vi "Test SaveToDisk.vi"(8 "error in (no error)":errorcluster, 11 "TestCase in":refnum<class "Verify IMemento.lvclass">) -> (0 "error out":errorcluster, 3 "TestCase out":refnum<class "Verify IMemento.lvclass">)   [LabVIEW 2009, in "Verify IMemento.lvclass"]
uses:
  Verify IMemento.lvclass
  Numeric Test Object/Interface Implementations/IMementoNumeric/MementoNumeric/MementoNumeric.lvclass
  Numeric Test Object/Numeric Test Object.lvclass
  Numeric Test Object/Interface Implementations/IMementoNumeric/IMementoNumeric.lvclass
  Framework Core/Interface Definitions/IMemento/IMemento.lvclass
  Verify IMemento.lvclass/Verify IMemento.ctl
  <vilib>/addons/_JKI Toolkits/VI Tester/TestCase.llb/TestCase.lvclass
  Source/Interfaceable Class/Interfaceable.lvclass
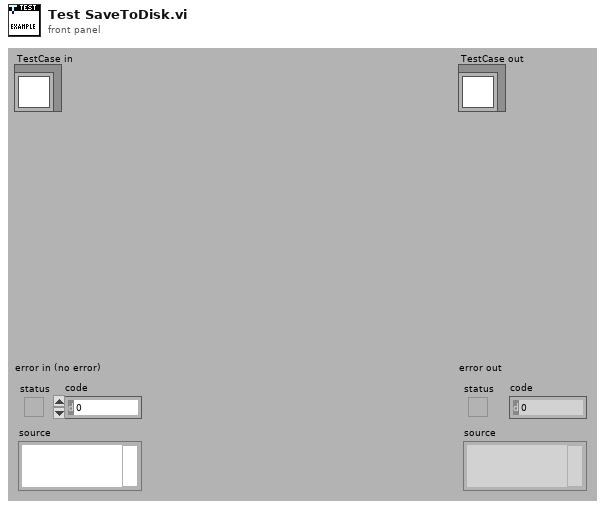
[diagram p1: front panel]
types:
  T1 = enum16{"open", "replace", "create", "open or create", "replace or create", "replace or create with confirmation"}
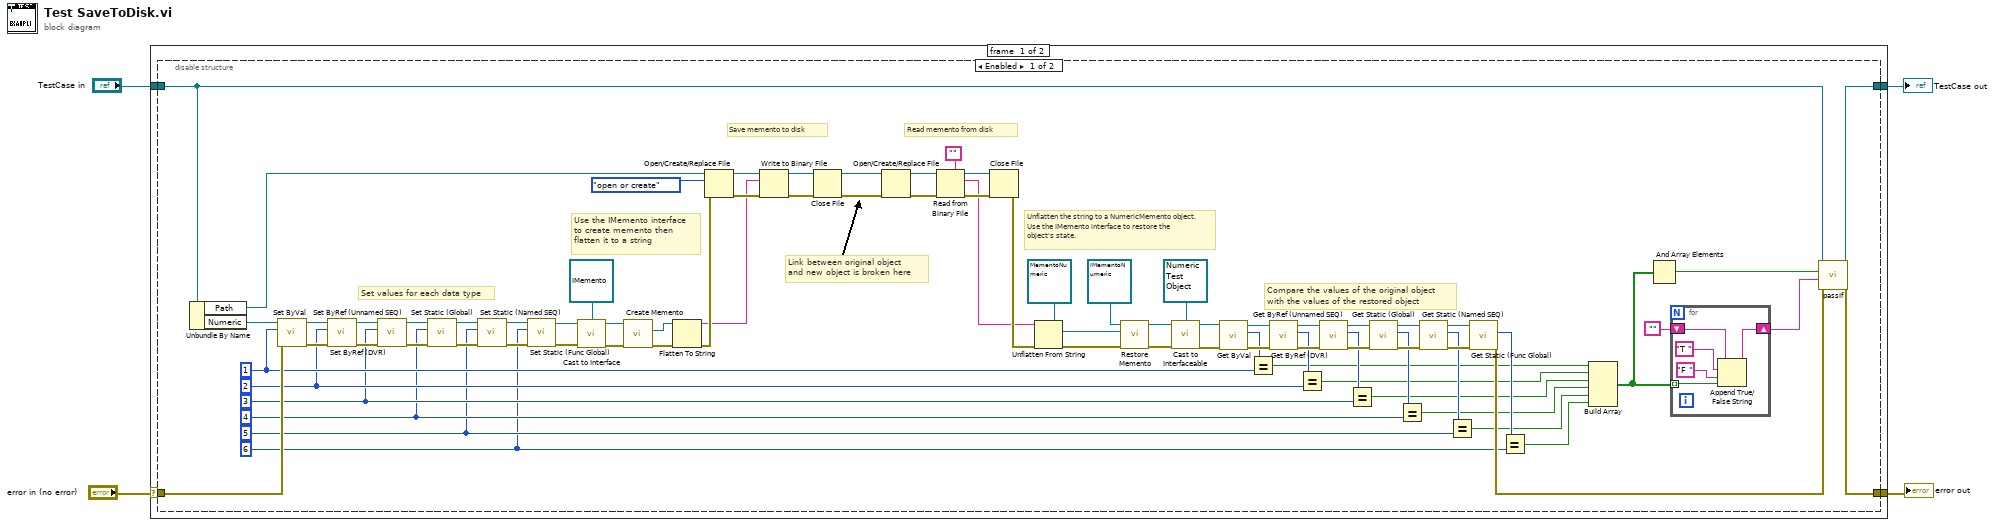
[diagram p0: block diagram]
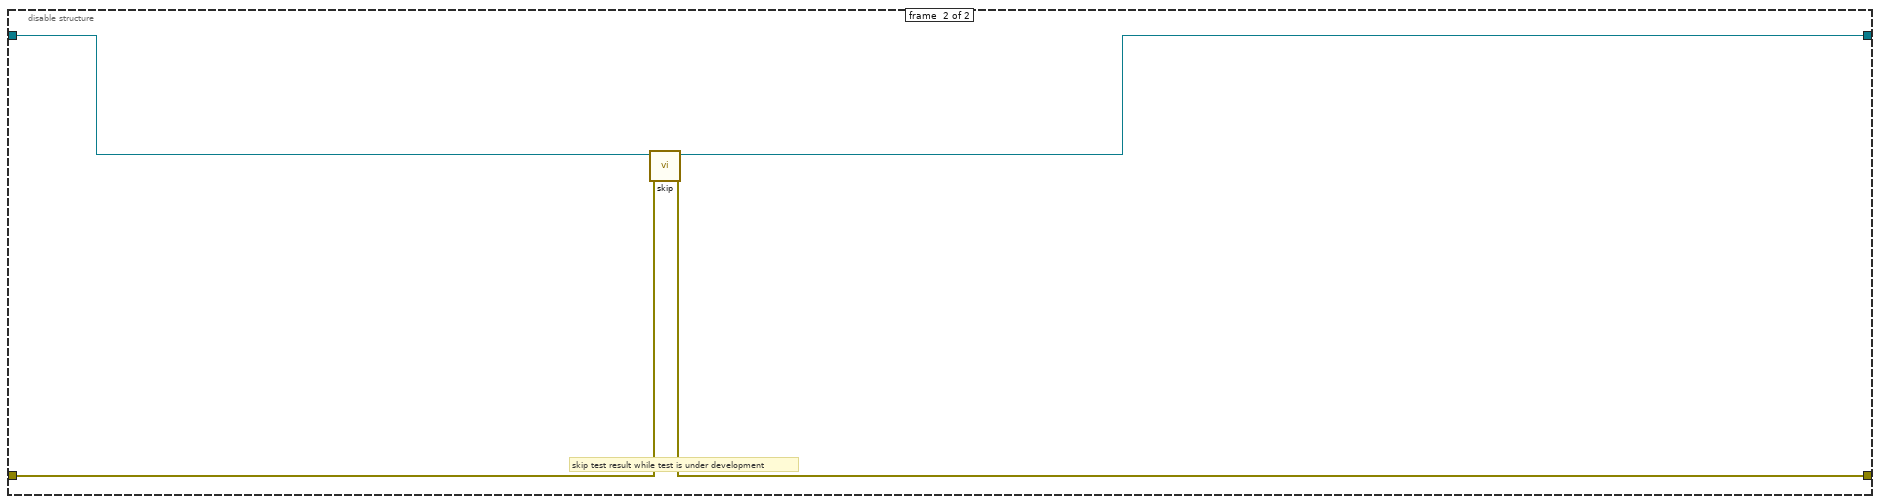
[diagram p2: hidden frame]
diagram:
  n1 = case shown="No Error" "error in (no error)" {
    selector: "error in (no error)" -> [w6 w100]
    tunnel: [w5 w100] -> w3
    tunnel: [w7 w99] -> w1
    tunnel: "TestCase in" -> [w8 w99]
    frame #0 {
      n2 = disable-structure shown="Enabled" {
        disable-tunnel: w8 -> [w66 w98]
        disable-tunnel: [w89 w95] -> w7
        disable-tunnel: w6 -> [w78 w97]
        disable-tunnel: [w88 w96] -> w5
        frame #0 {
          w29 = 1 ("Int")
          w27 = 2 ("Int")
          w25 = 3 ("Int")
          w23 = 4 ("Int")
          w21 = 5 ("Int")
          w19 = 6 ("Int")
          # "Link between original object and new object is broken here"
          # "Compare the values of the original object with the values of the restored object"
          # "Unflatten the string to a NumericMemento object. Use the IMemento interface to restore the object's state."
          # "Use the IMemento interface to create memento then flatten it to a string"
          # "Read memento from disk"
          # "Save memento to disk"
          # "Set values for each data type"
          n3 = Unbundle By Name(w66) -> ("Path"=w65:path, "Numeric"=w77:refnum<class "Numeric Test Object.lvclass">)
          n4 = call-dynamic "Set ByVal.vi"("error in (no error)"=w78, "Int"=w29, "Numeric in"=w77) -> ("error out"=w71:errorcluster, "Numeric out"=w76:refnum<class "Numeric Test Object.lvclass">)  [unwired: 7 in]
          n5 = call-dynamic "Set ByRef (DVR).vi"("error in (no error)"=w71, "Int"=w27, "Numeric in"=w76) -> ("error out"=w70:errorcluster, "Numeric out"=w75:refnum<class "Numeric Test Object.lvclass">)  [unwired: 7 in]
          n6 = call-dynamic "Set ByRef (Unnamed SEQ).vi"("error in (no error)"=w70, "Int"=w25, "Numeric in"=w75) -> ("error out"=w69:errorcluster, "Numeric out"=w74:refnum<class "Numeric Test Object.lvclass">)  [unwired: 7 in]
          n7 = call-dynamic "Set Static (Global).vi"("error in (no error)"=w69, "Int"=w23, "Numeric in"=w74) -> ("error out"=w68:errorcluster, "Numeric out"=w73:refnum<class "Numeric Test Object.lvclass">)  [unwired: 7 in]
          n8 = call-dynamic "Set Static (Named SEQ).vi"("error in (no error)"=w68, "Int"=w21, "Numeric in"=w73) -> ("error out"=w67:errorcluster, "Numeric out"=w72:refnum<class "Numeric Test Object.lvclass">)  [unwired: 7 in]
          n9 = call-dynamic "Set Static (Func Global).vi"("error in (no error)"=w67, "Int"=w19, "Numeric in"=w72) -> ("error out"=w86:errorcluster, "Numeric out"=w87:refnum<class "Numeric Test Object.lvclass">)  [unwired: 7 in]
          n10 = call "Cast to Interface.vi"("Target Interface"=refnum<class "IMemento.lvclass"> refnum ("IMemento"), "Interfaceable Object"=w87, "error in (no error)"=w86) -> ("Concrete Interface"=w84:refnum<class "IMemento.lvclass">, "error out"=w83:errorcluster)  [unwired: 5 in]
          n11 = call-dynamic "Create Memento.vi"("error in (no error)"=w83, "IMemento in"=w84) -> ("error out"=w53:errorcluster, "LabVIEW Object"=w51:refnum<class>)  [unwired: 7 in, 1 out]
          n12 = Flatten To String(anything=w51, error in (no error)=w53) -> (data string=w50:string, error out=w52:errorcluster)  [unwired: 2 in, 1 out]
          n13 = Open/Create/Replace File(file path (use dialog)=w65, error in=w52, operation (0:open)=T1."open or create") -> (refnum out=w63:refnum<file>, error out=w62:errorcluster)  [unwired: 3 in, 1 out]
          n14 = Write to Binary File(file (use dialog)=w63, data=w50, error in=w62) -> (refnum out=w61:refnum<file>, error out=w60:errorcluster)  [unwired: 3 in, 1 out]
          n15 = Close File(refnum=w61, error in=w60) -> (path=w59:path, error out=w58:errorcluster)
          n16 = Open/Create/Replace File(file path (use dialog)=w59, error in=w58) -> (refnum out=w57:refnum<file>, error out=w56:errorcluster)  [unwired: 4 in, 1 out]
          n17 = Read from Binary File(5:"" ("data type"), 8:w56, 11:w57) -> (0:w54:errorcluster, 2:w46:string, 3:w55:refnum<file>)  [unwired: 3 in, 1 out]
          n18 = Close File(refnum=w55, error in=w54) -> (error out=w48:errorcluster)  [unwired: 1 out]
          n19 = Unflatten From String(type=refnum<class "MementoNumeric.lvclass"> refnum ("MementoNumeric"), binary string=w46, error in (no error)=w48) -> (value=w43:refnum<class "MementoNumeric.lvclass">, error out=w47:errorcluster)  [unwired: 2 in, 1 out]
          n20 = call-dynamic "Restore Memento.vi"("error in (no error)"=w47, "Numeric Memento"=w43, "IMementoNumeric in"=refnum<class "IMementoNumeric.lvclass"> refnum ("IMementoNumeric")) -> ("error out"=w81:errorcluster, "IMementoNumeric out"=w82:refnum<class "IMementoNumeric.lvclass">)  [unwired: 7 in]
          n21 = call "Cast to Interfaceable.vi"("Target Object"=refnum<class "Numeric Test Object.lvclass"> refnum ("Numeric"), "Interface"=w82, "error in (no error)"=w81) -> ("Interfaceable Object"=w42:refnum<class "Numeric Test Object.lvclass">, "error out"=w41:errorcluster)  [unwired: 5 in]
          n22 = call-dynamic "Get ByVal.vi"("error in (no error)"=w41, "Numeric in"=w42) -> ("error out"=w35:errorcluster, "Int"=w30:i32, "Numeric out"=w40:refnum<class "Numeric Test Object.lvclass">)  [unwired: 7 in]
          n23 = Equal?(x=w30, y=w29) -> (x = y?=w18:bool)
          n24 = call-dynamic "Get ByRef (DVR).vi"("error in (no error)"=w35, "Numeric in"=w40) -> ("error out"=w34:errorcluster, "Int"=w28:i32, "Numeric out"=w39:refnum<class "Numeric Test Object.lvclass">)  [unwired: 7 in]
          n25 = Equal?(x=w28, y=w27) -> (x = y?=w17:bool)
          n26 = call-dynamic "Get ByRef (Unnamed SEQ).vi"("error in (no error)"=w34, "Numeric in"=w39) -> ("error out"=w33:errorcluster, "Int"=w26:i32, "Numeric out"=w38:refnum<class "Numeric Test Object.lvclass">)  [unwired: 7 in]
          n27 = Equal?(x=w26, y=w25) -> (x = y?=w16:bool)
          n28 = call-dynamic "Get Static (Global).vi"("error in (no error)"=w33, "Numeric in"=w38) -> ("error out"=w32:errorcluster, "Int"=w24:i32, "Numeric out"=w37:refnum<class "Numeric Test Object.lvclass">)  [unwired: 7 in]
          n29 = Equal?(x=w24, y=w23) -> (x = y?=w15:bool)
          n30 = call-dynamic "Get Static (Named SEQ).vi"("error in (no error)"=w32, "Numeric in"=w37) -> ("error out"=w31:errorcluster, "Int"=w22:i32, "Numeric out"=w36:refnum<class "Numeric Test Object.lvclass">)  [unwired: 7 in]
          n31 = Equal?(x=w22, y=w21) -> (x = y?=w14:bool)
          n32 = call-dynamic "Get Static (Func Global).vi"("error in (no error)"=w31, "Numeric in"=w36) -> ("error out"=w79:errorcluster, "Int"=w20:i32)  [unwired: 7 in, 1 out]
          n33 = Equal?(x=w20, y=w19) -> (x = y?=w13:bool)
          n34 = Build Array(w18, w17, w16, w15, w14, w13) -> (w10:bool[])
          n35 = And Array Elements(Boolean array=w10) -> (logical AND=w12:bool)
          n36 = for {
            tunnel: w10 -> [w94] mode=indexing
            shift-right: [w93] -> w9
            shift-left: "" -> [w90]
            n37 = Append True/False String(1:w94, 2:"F " ("false string"), 3:"T " ("true string"), 4:w90) -> (0:w93:string)
          }
          n38 = call-dynamic "passIf.vi"("error in (no error)"=w79, "message (\"\")"=w9, "pass"=w12, "TestCase in"=w66) -> ("error out"=w88:errorcluster, "TestCase out"=w89:refnum<class "Verify IMemento.lvclass">)  [unwired: 6 in]
        }
        frame #1 {
          # "skip test result while test is under development"
          n39 = call <vilib>:"skip.vi"("error in (no error)"=w97, "TestCase in"=w98) -> ("error out"=w96:errorcluster, "TestCase out"=w95:refnum<class "Verify IMemento.lvclass">)  [unwired: 8 in]
        }
      }
    }
    frame #1 {
    }
  }
  "error out" <- w3
  "TestCase out" <- w1
